vi "Alarms.SetAll.vi"(8 "error in (no error)":errorcluster, 10 "Alarms":T1[](array[typedef]) {"Delay" format="%.2f"; "Low Limit" format="%.2f"; "High Limit" format="%.2f"}, 11 "ListBox in":refnum<vi>) -> (0 "error out":errorcluster)   [LabVIEW 2015, in "Single Station Execution.lvlib"]
uses:
  Single Station Execution.lvlib
  Types/Config.AlarmSettings.ctl
  <vilib>/NI Veristand/Execution/Alarm/NI_VS Alarm ExecutionAPI.lvlib
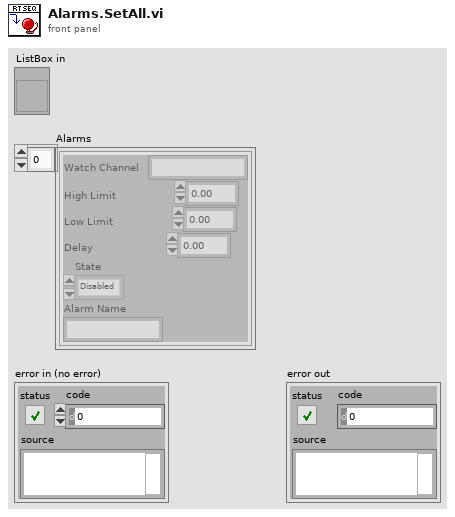
[diagram p1: front panel]
types:
  T1 = typedef "Single Station Execution.lvlib/Config.AlarmSettings.ctl" = cluster{"Watch Channel":string, "High Limit":dbl, "Low Limit":dbl, "Delay":dbl, "State":enum16{"Disabled", "Enabled", "Tripped", "Delayed Trip", "Indicate"}, "Alarm Name":string}
  T2 = enum16{"Disabled", "Enabled", "Tripped", "Delayed Trip", "Indicate"}
  T3 = typedef "NI_VS Alarm ExecutionAPI.lvlib/AlarmAPI.ctl" = refnum<k24>
  T4 = typedef "NI_VS Alarm ExecutionAPI.lvlib/AlarmInfo.ctl" = cluster{"Watch Channel":string, "High Limit Constant":bool, "High Limit Channel":string, "High Limit":dbl, "Low Limit Constant":bool, "Low Limit Channel":string, "Low Limit":dbl, "Procedure Name":string, "Delay":dbl, "Trip Value":dbl, "Priority":enum16{"Low", "Medium", "High"}, "State":enum16{"Disabled", "Enabled", "Tripped", "Delayed Trip", "Indicate"}, "Mode":enum16{"Normal", "Indicate Only"}, "Group Number":u32, "Priority Number":u32, "Name":string, "Full Name":string}
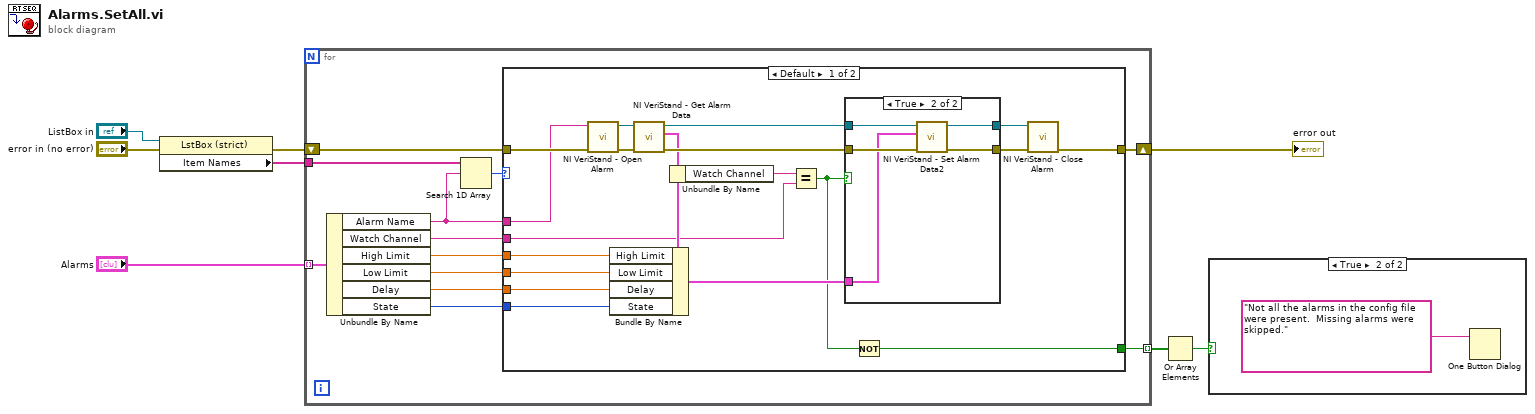
[diagram p0: block diagram]
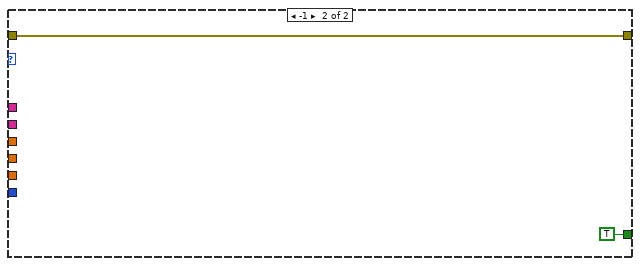
[diagram p4: hidden frame]
diagram:
  n1 = property class="LstBox (strict)"(reference="ListBox in", error in="error in (no error)") -> (error out=w3:errorcluster, "Item Names"=w5:string[])  [unwired: 1 out]
  n2 = for {
    shift-right: [w16] -> w6
    shift-left: w3 -> [w17]
    tunnel: "Alarms" -> [w20] mode=indexing
    tunnel: w5 -> [w19]
    tunnel: [w9] -> w7 mode=indexing
    n3 = Unbundle By Name(w20) -> ("Alarm Name"=w15:string, "Watch Channel"=w10:string, "High Limit"=w11:dbl, "Low Limit"=w12:dbl, "Delay"=w13:dbl, "State"=w14:T2)
    n4 = Search 1D Array(1D array=w19, element=w15) -> (index of element=w18:i32)  [unwired: 1 in]
    n5 = case shown="Default" w18 {
      tunnel: w17 -> [w39 w48]
      tunnel: [w35 w48] -> w16
      tunnel: w15 -> [w24 _]
      tunnel: w14 -> [w29 _]
      tunnel: w13 -> [w28 _]
      tunnel: w12 -> [w27 _]
      tunnel: w11 -> [w26 _]
      tunnel: w10 -> [w25 _]
      tunnel: [w21 TRUE] -> w9
      frame Default {
        n6 = call <vilib>:"NI VeriStand - Open Alarm.vi"("error in (no error)"=w39, "Alarm Name"=w24) -> ("error out"=w38:errorcluster, "Alarm"=w34:T3)  [unwired: 8 in]
        n7 = call <vilib>:"NI VeriStand - Get Alarm Data.vi"("error in (no error)"=w38, "Alarm in"=w34) -> ("error out"=w37:errorcluster, "Alarm Data"=w30:T4, "Alarm out"=w33:T3)  [unwired: 7 in]
        n8 = Bundle By Name(cluster=w30, "High Limit"=w26, "Low Limit"=w27, "Delay"=w28, "State"=w29) -> (w23:T4)
        n9 = Unbundle By Name(w30) -> ("Watch Channel"=w31:string)
        n10 = Equal?(x=w31, y=w25) -> (x = y?=w22:bool)
        n11 = case shown="True" w22 {
          tunnel: w37 -> [w41 w46]
          tunnel: [w41 w45] -> w36
          tunnel: w33 -> [w40 w44]
          tunnel: [w40 w43] -> w32
          tunnel: w23 -> [_ w42]
          frame False {
          }
          frame True {
            n12 = call <vilib>:"NI VeriStand - Set Alarm Data2.vi"("error in (no error)"=w46, "Alarm Data"=w42, "Alarm in"=w44) -> ("error out"=w45:errorcluster, "Alarm out"=w43:T3)  [unwired: 7 in]
          }
        }
        n13 = Not(x=w22) -> (.not. x?=w21:bool)
        n14 = call <vilib>:"NI VeriStand - Close Alarm.vi"("error in (no error)"=w36, "Alarm"=w32) -> ("error out"=w35:errorcluster)  [unwired: 9 in]
      }
      frame -1 {
      }
    }
  }
  "error out" <- w6
  n15 = Or Array Elements(Boolean array=w7) -> (logical OR=w8:bool)
  n16 = case shown="True" w8 {
    frame False {
    }
    frame True {
      n17 = One Button Dialog(message="Not all the alarms in the config file were present.  Missing alarms were skipped.") -> ()  [unwired: 1 in, 1 out]
    }
  }
